vi "TCP Engine Send Commands To all Modules.vi"(6 "Main Engine Command Q":refnum<queue>, 7 "Active Engine Names":string[](array[string]), 8 "error in":errorcluster, 9 "Engine Name":string[](array[string]), 10 "TCP Engine Log File Path":path, 11 "JSON String":string) -> (0 "error out":errorcluster, 3 "Active Engine Names Out":string[](array[string]))   [LabVIEW 2024, in "TCP Engine.lvlib"]
doc: "The purpose of this VI is to perform all functions of the hardware modules.\nFunctions\n1)Engine Launch\n2)Configuration\n3)Update\n4)All Start\n5)Engine start\n6)Hardware Info.\n\n\nAll Rights Reserved © 2017 SyncSols"
uses:
  TCP Engine.lvlib
  Main Engine/Controls/Main Engine Command Cluster.ctl
  Main Engine/Controls/Main Engine TCP Command Data.ctl
  Analog Output/Controls/AO JSON Data Cluster.ctl
  Analog Output/Controls/AO Interface Data Cluster.ctl
  Analog Output/Controls/AO Channel Configuration Cluster.ctl
  Analog Output/Controls/AO Timing Cluster.ctl
  Analog Output/Controls/AIO Command Q Cluster.ctl
  Main Engine/Controls/Main Engine JSON Command State.ctl
  Controls/TCP Engine I&O  Interupt Cluster.ctl
  Analog Output/Controls/AO 1D DBL ArrayCluster.ctl
  Analog Output/Controls/AO 1D DBL Interface Data Cluster.ctl
  Analog Output/Controls/AO DBL Data Cluster.ctl
  Digital Output/Controls/DIO Configuration cluster.ctl
  Digital Output/Controls/DIO Interface Data.ctl
  Digital Output/SubVIs/Digital Dynamic Cluster.ctl
  Digital Output/Controls/DIO Commad Q Cluster.ctl
  Digital Output/Controls/DO Update Cluster.ctl
  Async Serial/Controls/Async Serial Command Q Cluster.ctl
  Async Serial/Controls/Async Serial Configuration Cluster.ctl
  Async Serial/Controls/Async Frame Info Cluster.ctl
  Async Serial/Controls/Async Message Info Cluster.ctl
  Controls/TCP Engine Serial Interupt Cluster.ctl
  Async Serial/Controls/Async Update Cluster.ctl
  Async Serial/Controls/Async Waveform Config Cluster.ctl
  Analog Output/Controls/AO Sampling Info Cluster.ctl
  Ethernet/Controls/Ethernet Command Q Cluster.ctl
  Ethernet/Controls/Ethernet Configuration Cluster.ctl
  Ethernet/Controls/Ethernet Frame Info Cluster.ctl
  Ethernet/Controls/Ethernet Message Info Cluster.ctl
  Ethernet/Controls/Ethernet Dynamic Data Cluster.ctl
  Ethernet/Controls/Ethernet Update Cluster.ctl
  Controls/TCP Engine Q Driver Options.ctl
  Controls/TCP Engine State Machine Cases.ctl
  <vilib>/Utility/error.llb/Error Cluster From Error Code.vi
  <vilib>/ErrorRing/Error Ring.xnode
  <vilib>/addons/_JKI.lib/Serialization/JSON/JKI JSON Serialization.lvlib
  RT-DQMH-Module's/RT-AutoSequence/RT-AutoSequence.lvlib
  RT-DQMH-Module's/RT-TDMS-Logging/RT-TDMS-Logging.lvlib
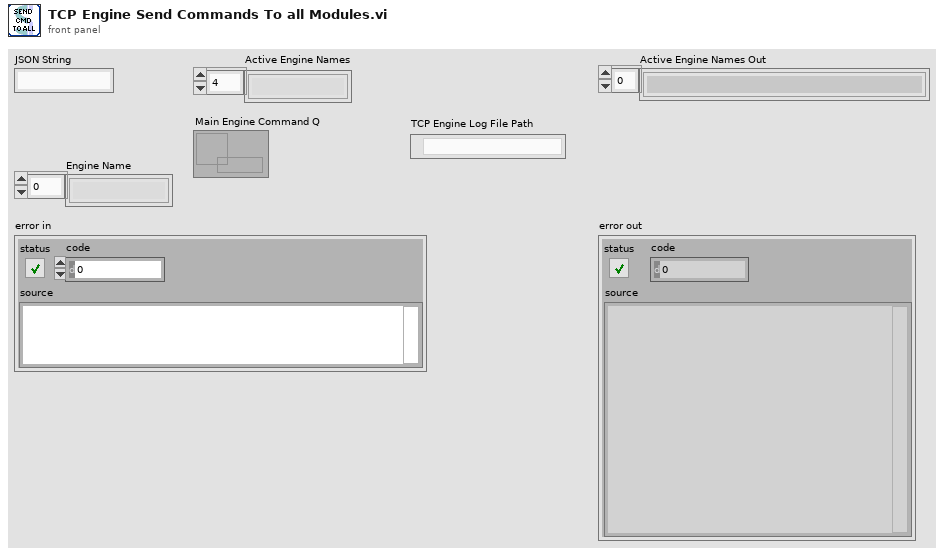
[diagram p1: front panel]
types:
  T1 = typedef "Main Engine TCP Command Data.ctl" = enum16{"Get HW Info", "Launch Module", "Get CPU Load", "Close CPU Load", "Exit"}
  T2 = typedef "Main Engine Command Cluster.ctl" = cluster{"State":T1, "Interface":string, "Engine Name":string, "Varient Data":variant, "SubCmd":string, "Serial Mode":string, "ARINC Board":u8, "Ethernet Mode":u8, "CPU Frequency":dbl}
  T3 = typedef "Main Engine JSON Command State.ctl" = enum16{"Configure", "Start", "Exit"}
  T4 = typedef "AO JSON Data Cluster.ctl" = cluster{"Interface":string, "Interface Data":T5}
  T5 = typedef "AO Interface Data Cluster.ctl" = cluster{"Command":string, "SubCmd":string, "Data":T6[], "Timing":T7}
  T6 = typedef "AO Channel Configuration Cluster.ctl" = cluster{"Channel":string, "Min Value":dbl, "Max Value":dbl, "Type":string, "Terminal Configure":u16, "Dynamic":u8, "Dyn Type":string, "Data":dbl[], "File Name":string, "Column":i32, "Frequency":dbl}
  T7 = typedef "AO Timing Cluster.ctl" = cluster{"samples per channel":i32, "sample mode":i32, "Sampling Rate":dbl}
  T8 = typedef "AIO Command Q Cluster.ctl" = cluster{"Interface":string, "Interface Data":T5, "Command State":T3}
  T9 = typedef "AO 1D DBL ArrayCluster.ctl" = cluster{"Interface":string, "Interface Data":T10}
  T10 = typedef "AO 1D DBL Interface Data Cluster.ctl" = cluster{"Command":string, "SubCmd":string, "Data":T11[]}
  T11 = typedef "AO DBL Data Cluster.ctl" = cluster{"Channel":string, "Data":dbl}
  T12 = typedef "DIO Commad Q Cluster.ctl" = cluster{"Interface":string, "Interface Data":cluster{"Command":string, "SubCmd":string, "Frequency":u16, "Data":T13[]}, "Command State":T3, "Data":variant}
  T13 = typedef "Digital Dynamic Cluster.ctl" = cluster{"Channel":string, "Data":u8[], "Identification Name":string}
  T14 = typedef "DO Update Cluster.ctl" = cluster{"Channel":string[], "Data":u8[]}
  T15 = typedef "Async Serial Configuration Cluster.ctl" = cluster{"Port":string, "Minor Frame Freq":u16, "Minor Frame Count":u16, "Frame Info":T16[], "Sensor Type":u16, "OIM Address":u16}
  T16 = typedef "Async Frame Info Cluster.ctl" = cluster{"Frame ID":u16, "Message Info":T17[]}
  T17 = typedef "Async Message Info Cluster.ctl" = cluster{"Message":u8[], "Message Name":string}
  T18 = typedef "Async Serial Command Q Cluster.ctl" = cluster{"Async serial Configuration Cluster":T15, "Command State":T3}
  T19 = typedef "Async Update Cluster.ctl" = cluster{"Port":string, "Message Info":T17[]}
  T20 = typedef "Async Waveform Config Cluster.ctl" = cluster{"Port":string, "Pattern":string, "Amplitude":dbl, "Frequency":dbl, "Phase":i32, "Sampling info":T21}
  T21 = typedef "AO Sampling Info Cluster.ctl" = cluster{"Fs":dbl, "#s":dbl}
  T22 = typedef "Ethernet Configuration Cluster.ctl" = cluster{"Mode":u8, "Local IP":string, "Local Port":u16, "Frame Info":T23[], "Minor Frame Freq":u8}
  T23 = typedef "Ethernet Frame Info Cluster.ctl" = cluster{"Frame ID":u16, "Message Info":T24[]}
  T24 = typedef "Ethernet Message Info Cluster.ctl" = cluster{"Message":u8[], "Message Name":string, "Dynamic":u8, "DynData":T25[], "Client IP":string, "Client Port":u16}
  T25 = typedef "Ethernet Dynamic Data Cluster.ctl" = cluster{"Type":string, "Start Byte":u8, "End Byte":u8, "Data":u32[][], "File Name":string, "Column":i32}
  T26 = typedef "Ethernet Command Q Cluster.ctl" = cluster{"Ethernet Configuration":T22, "Command State":T3}
  T27 = typedef "Ethernet Update Cluster.ctl" = cluster{"IP":string, "Message Info":T17[], "Port":u16}
  T28 = typedef "TCP Engine.lvlib/TCP Engine Q Driver Options.ctl" = enum16{"Initialize", "EnQ", "DeQ", "EnQ at Opp", "Get Q Status", "Flush Q", "Release Q"}
  T29 = typedef "TCP Engine.lvlib/TCP Engine I&O  Interupt Cluster.ctl" = cluster{" Stop":bool, "JSON Variant":variant}
  T30 = typedef "DIO Configuration cluster.ctl" = cluster{"Interface":string, "Interface Data":T31}
  T31 = typedef "DIO Interface Data.ctl" = cluster{"Command":string, "SubCmd":string, "Frequency":u16, "Data":T13[]}
  T32 = typedef "TCP Engine.lvlib/TCP Engine Serial Interupt Cluster.ctl" = cluster{"Stop":bool, "JSON Variant":variant}
  T33 = typedef "TCP Engine.lvlib/TCP Engine State Machine Cases.ctl" = enum16{">Poll", ".........State Machine.........", ">Init", ">Init Configuration", ">Decode Configuration", ">Error", ">Exit", "..........TCP Engine..........", ">Wait for Listener", ">Get Msg from HOST", ">Decode the Command", ">Create Listerner ID"}
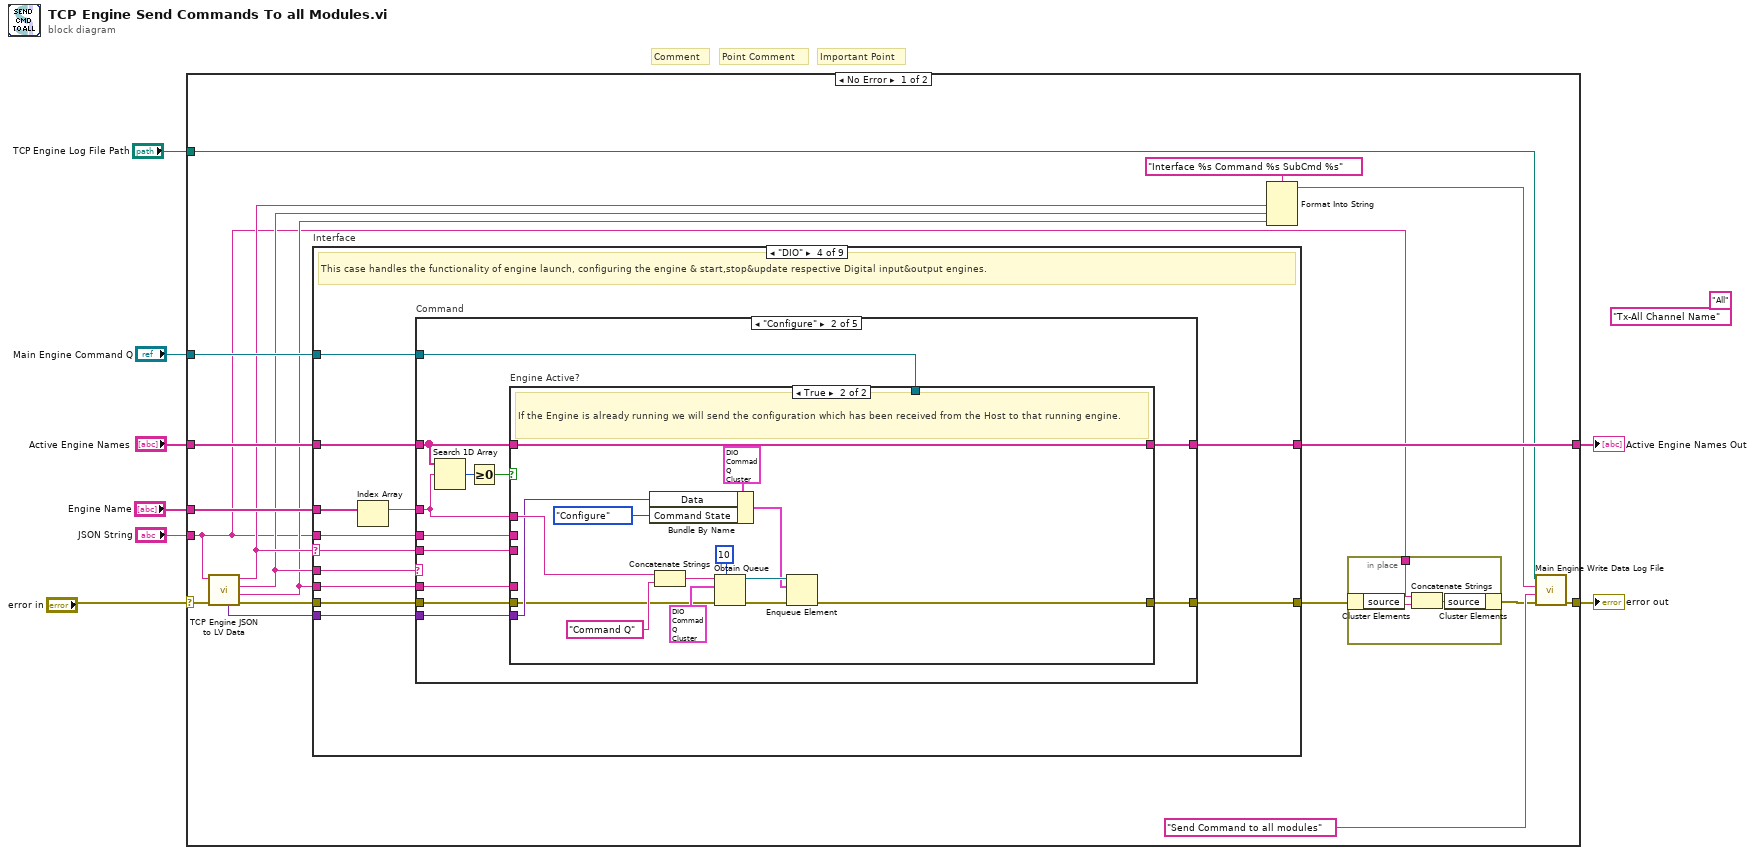
[diagram p0: block diagram]
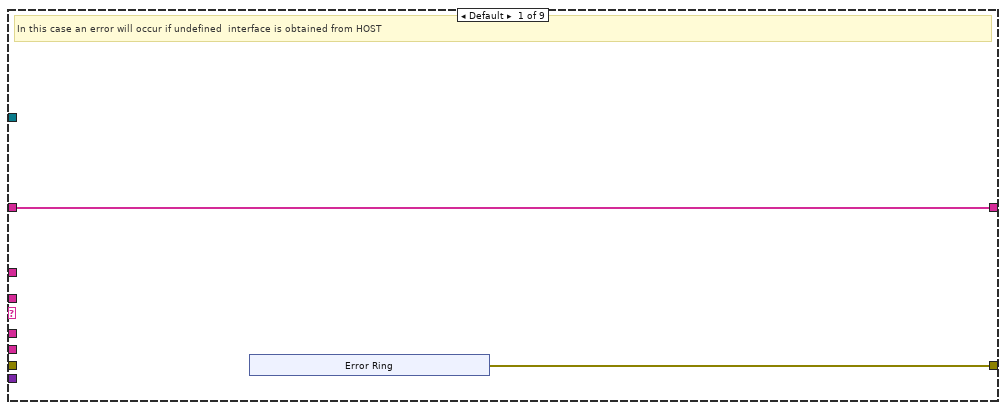
[diagram p2: hidden frame]
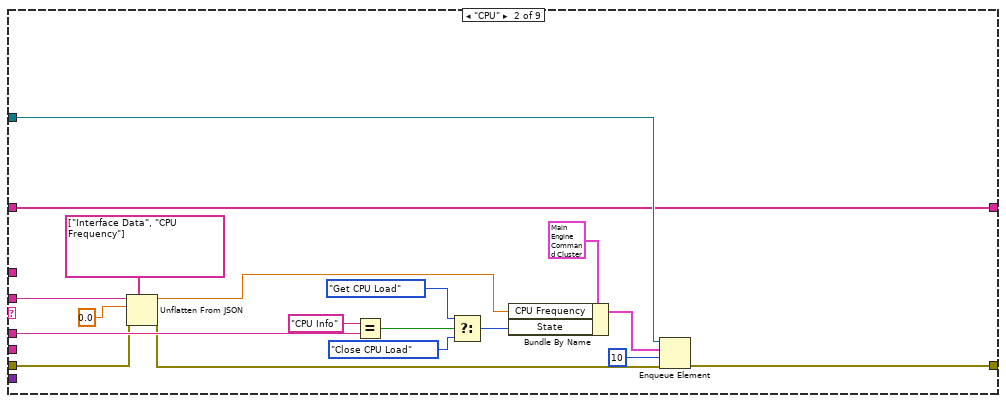
[diagram p3: hidden frame]
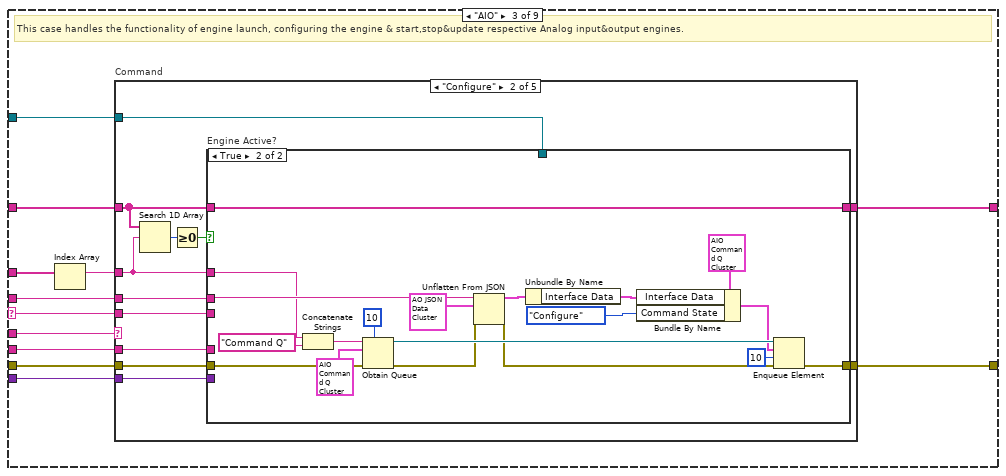
[diagram p4: hidden frame]
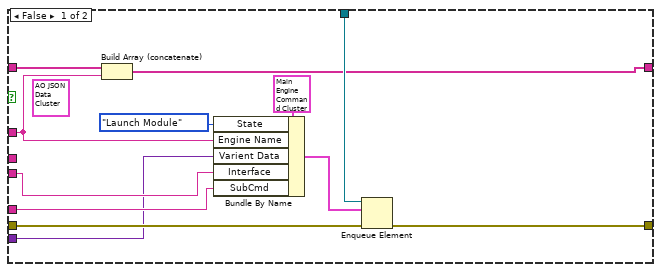
[diagram p6: hidden frame]
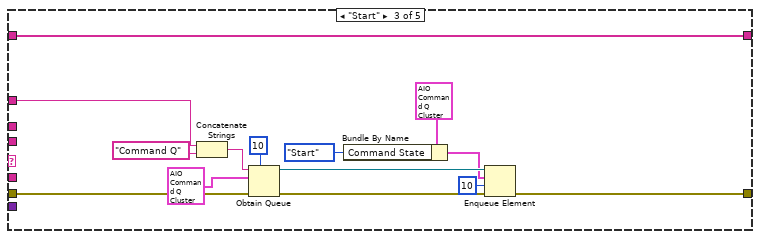
[diagram p7: hidden frame]
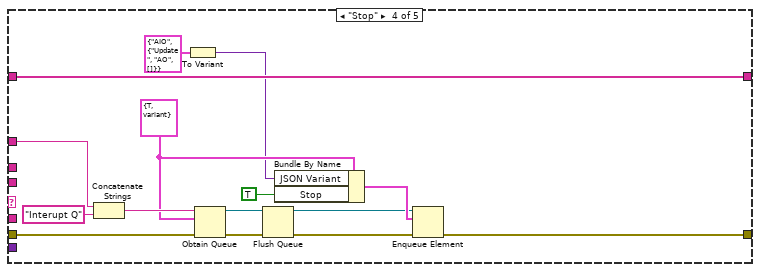
[diagram p8: hidden frame]
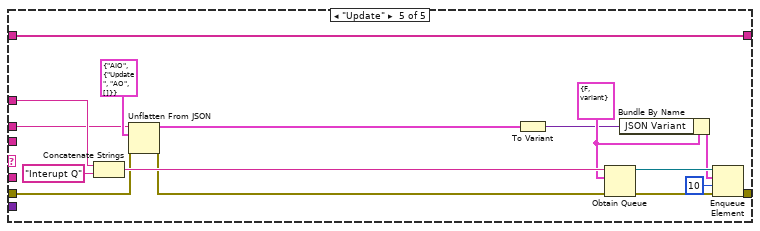
[diagram p9: hidden frame]
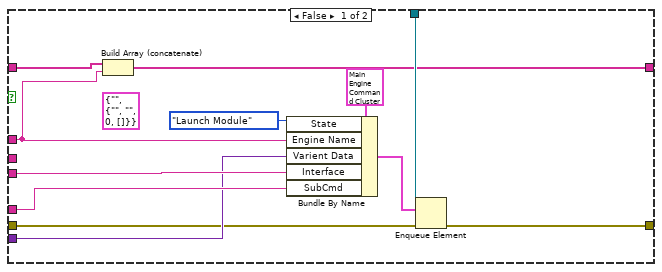
[diagram p11: hidden frame]
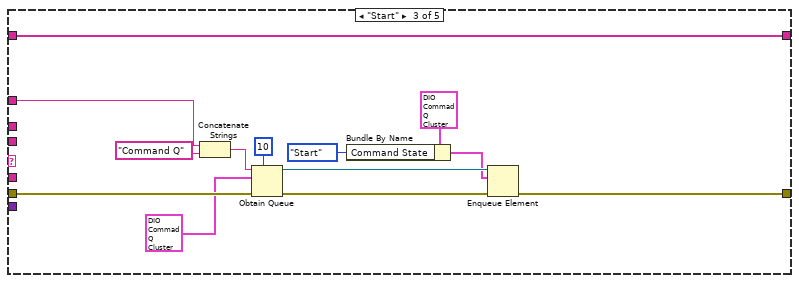
[diagram p12: hidden frame]
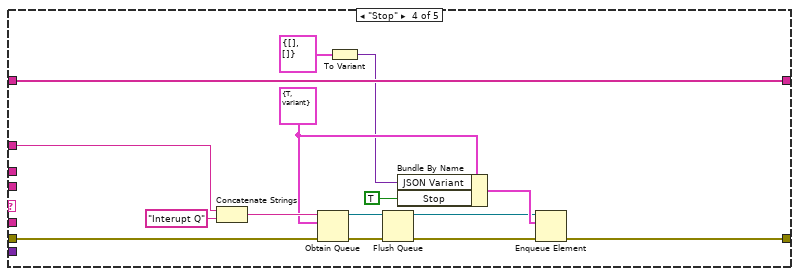
[diagram p13: hidden frame]
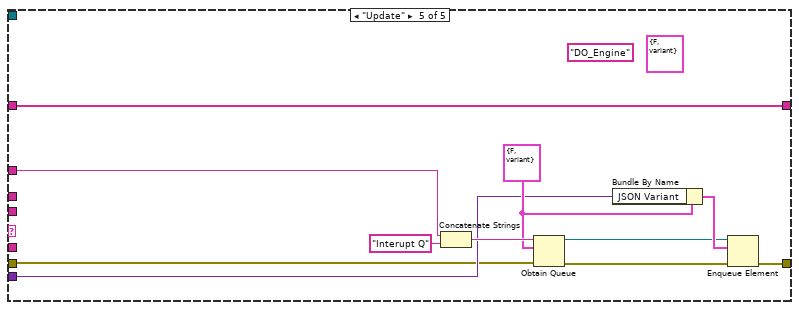
[diagram p14: hidden frame]
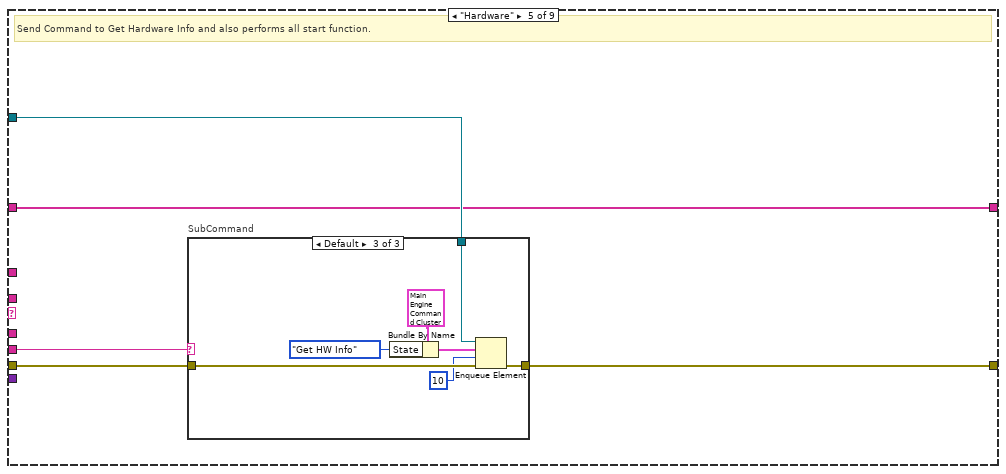
[diagram p15: hidden frame]
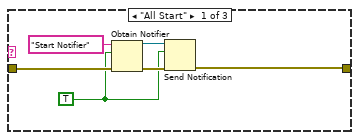
[diagram p16: hidden frame]
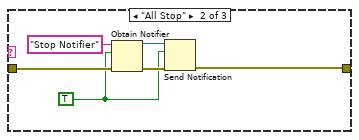
[diagram p17: hidden frame]
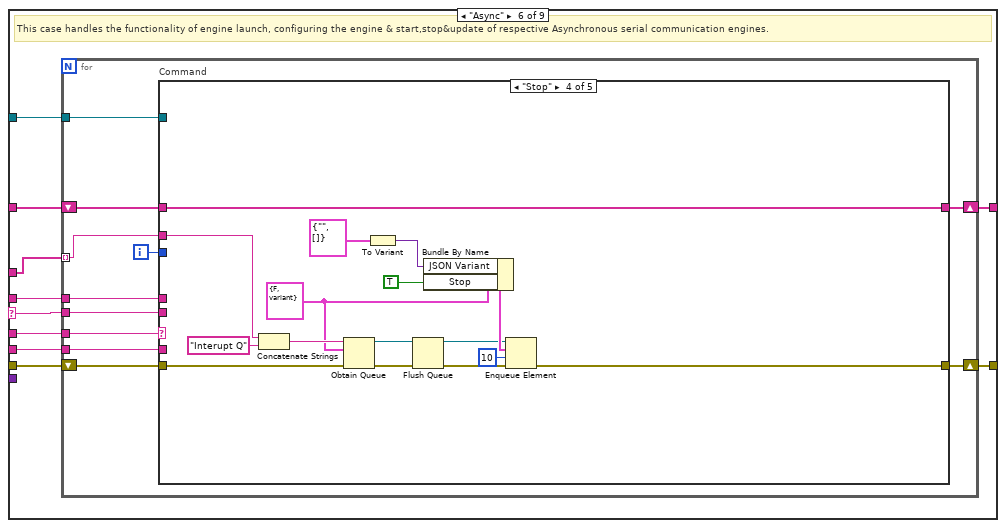
[diagram p18: hidden frame]
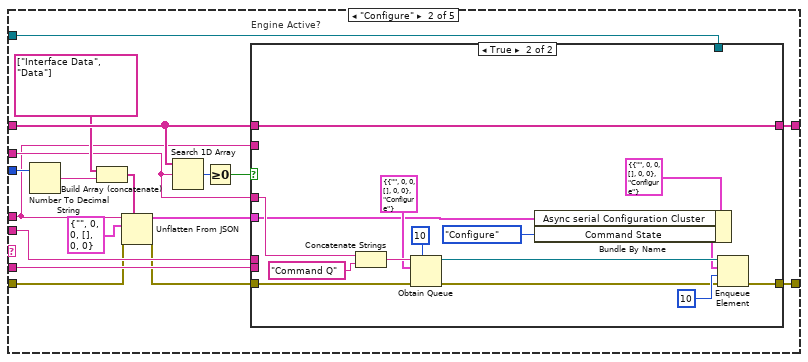
[diagram p20: hidden frame]
diagram:
  (unwired) "Tx-All Channel Name" ("Interface Data.Command")
  (unwired) "All" ("Interface")
  # "Important Point"
  # "Point Comment"
  # "Comment"
  n1 = case shown="No Error" "error in" {
    selector: "error in" -> [w24 w610]
    tunnel: [w20 w612] -> w8
    tunnel: "Engine Name" -> [w22 _]
    tunnel: "JSON String" -> [w10 w609]
    tunnel: "Main Engine Command Q" -> [w26 _]
    tunnel: "Active Engine Names" -> [w25 w613]
    tunnel: [w21 w613] -> w3
    tunnel: "TCP Engine Log File Path" -> [w14 w611]
    frame No Error {
      n2 = call "TCP Engine JSON to LV Data.vi"("error in"=w24, "Cmd String"=w10) -> ("error out"=w23:errorcluster, "SubCmd"=w16:string, "Command"=w17:string, "Interface"=w18:string, "Data"=w9:variant)  [unwired: 4 in, 1 out]
      n3 = case "Interface" shown="\"DIO\"" w18 {
        selector: w18 -> [_ _ w58 w160 _ w276 w421 _ _]
        tunnel: [w31 w54 w64 w166 w250 w281 w426 w548 w579] -> w12
        tunnel: w23 -> [_ w42 w66 w168 w252 w274 w419 w544 w578]
        tunnel: w26 -> [_ w53 w65 w167 w251 w279 w424 _ _]
        tunnel: w22 -> [_ _ w63 w165 _ w275 w420 _ _]
        tunnel: w10 -> [_ w40 w62 w164 _ w273 w418 _ _]
        tunnel: w25 -> [w30 w43 w60 w162 w249 w278 w423 w545 w581]
        tunnel: w17 -> [_ w49 w61 w163 _ w272 w417 _ w580]
        tunnel: w16 -> [_ _ w59 w161 w248 w277 w422 _ w577]
        tunnel: [w30 w43 w57 w159 w249 w280 w425 w545 w581] -> w21
        tunnel: w9 -> [_ _ w55 w157 _ _ _ _ w576]
        frame Default {
          # "In this case an error will occur if undefined  interface is obtained from HOST"
          n4 = xnode "Error Ring"() -> ("error out"=w31:errorcluster)
        }
        frame "CPU" {
          n5 = Unflatten From JSON(path=string[] ["Interface Data", "CPU Frequency"], JSON string=w40, type and defaults=0.0, error in (no error)=w42) -> (value=w37:dbl, error out=w41:errorcluster)  [unwired: 3 in]
          n6 = Equal?(x="CPU Info", y=w49) -> (x = y?=w47:bool)
          n7 = Select(t=Main_Engine_TCP_Command_Data."Get CPU Load" ("State"), s=w47, f=Main_Engine_TCP_Command_Data."Close CPU Load" ("State")) -> (s? t:f=w44:T1)
          n8 = Bundle By Name(cluster=T2 {"State"=enum."Launch Module", "Interface"="AO", "Engine Name"="Slot5_6551_AO", "Varient Data"=variant(string "{"), "SubCmd"="", "Serial Mode"="", "ARINC Board"=0, "Ethernet Mode"=0, "CPU Frequency"=0.0}, "CPU Frequency"=w37, "State"=w44) -> (w50:T2)
          n9 = Enqueue Element(queue=w53, element=w50, timeout in ms (-1)=10, error in (no error)=w41) -> (error out=w54:errorcluster)  [unwired: 2 out]
        }
        frame "AIO" {
          # "This case handles the functionality of engine launch, configuring the engine & start,stop&update respective Analog input&output engines."
          n10 = Index Array(array=w63) -> (element=w56:string)  [unwired: 1 in]
          n11 = case "Command" shown="\"Configure\"" w61 {
            tunnel: w66 -> [w68 w80 w125 w140 w146]
            tunnel: w65 -> [_ w79 _ _ _]
            tunnel: [w68 w78 w124 w133 w149] -> w64
            tunnel: w56 -> [_ w70 w123 w138 w155]
            tunnel: w62 -> [_ w77 _ _ w144]
            tunnel: w60 -> [w67 w72 w112 w132 w148]
            tunnel: w59 -> [_ w74 _ _ _]
            tunnel: w58 -> [_ w73 _ _ _]
            tunnel: [w67 w71 w112 w132 w148] -> w57
            tunnel: w55 -> [_ w69 _ _ _]
            frame Default {
            }
            frame "Configure" {
              n12 = Search 1D Array(1D array=w72, element=w70) -> (index of element=w76:i32)  [unwired: 1 in]
              n13 = Greater Or Equal To 0?(x=w76) -> (x >= 0?=w75:bool)
              n14 = case "Engine Active?" shown="True" w75 {
                tunnel: w80 -> [w92 w111]
                tunnel: w79 -> [w91 _]
                tunnel: [w90 w110] -> w78
                tunnel: w77 -> [_ w95]
                tunnel: w74 -> [w83 _]
                tunnel: w73 -> [w86 _]
                tunnel: w72 -> [w85 w93]
                tunnel: [w84 w93] -> w71
                tunnel: w70 -> [w82 w94]
                tunnel: w69 -> [w81 _]
                frame False {
                  (unwired) T4 {"Interface"="AIO", "Interface Data"={"Command"="Configure", "SubCmd"="AO", "Data"=[], "Timing"={"samples per channel"=0, "sample mode"=10178, "Sampling Rate"=0.0}}} ("AO JSON Data Cluster")
                  n15 = Build Array (concatenate)(w85, w82) -> (w84:string[])
                  n16 = Bundle By Name(cluster=T2 {"State"=enum."Launch Module", "Interface"="AO", "Engine Name"="Slot5_6551_AO", "Varient Data"=variant(string "{"), "SubCmd"="", "Serial Mode"="", "ARINC Board"=0, "Ethernet Mode"=0, "CPU Frequency"=0.0}, "State"=Main_Engine_TCP_Command_Data."Launch Module", "Engine Name"=w82, "Varient Data"=w81, "Interface"=w86, "SubCmd"=w83) -> (w88:T2)
                  n17 = Enqueue Element(queue=w91, element=w88, error in (no error)=w92) -> (error out=w90:errorcluster)  [unwired: 1 in, 2 out]
                }
                frame True {
                  n18 = Concatenate Strings(w94, "Command Q" ("string")) -> (w109:string)
                  n19 = Obtain Queue(max queue size (-1, unlimited)=10, name (unnamed)=w109, element data type=T8 {"Interface"="AIO", "Interface Data"={"Command"="Configure", "SubCmd"="AO", "Data"=[], "Timing"={"samples per channel"=1000, "sample mode"=10178, "Sampling Rate"=1000.0}}, "Command State"=enum."Configure"}, error in (no error)=w111) -> (queue out=w107:refnum<queue>, error out=w97:errorcluster)  [unwired: 1 in, 1 out]
                  n20 = Unflatten From JSON(JSON string=w95, type and defaults=T4 {"Interface"="AIO", "Interface Data"={"Command"="Configure", "SubCmd"="AO", "Data"=[], "Timing"={"samples per channel"=1000, "sample mode"=10178, "Sampling Rate"=1000.0}}}, error in (no error)=w97) -> (value=w101:T4, error out=w96:errorcluster)  [unwired: 4 in]
                  n21 = Unbundle By Name(w101) -> ("Interface Data"=w100:T5)
                  n22 = Bundle By Name(cluster=T8 {"Interface"="AIO", "Interface Data"={"Command"="Configure", "SubCmd"="AO", "Data"=[], "Timing"={"samples per channel"=1000, "sample mode"=10178, "Sampling Rate"=1000.0}}, "Command State"=enum."Configure"}, "Interface Data"=w100, "Command State"=Main_Engine_JSON_Command_State."Configure") -> (w98:T8)
                  n23 = Enqueue Element(queue=w107, element=w98, timeout in ms (-1)=10, error in (no error)=w96) -> (error out=w110:errorcluster)  [unwired: 2 out]
                }
              }
            }
            frame "Start" {
              n24 = Concatenate Strings(w123, "Command Q" ("string")) -> (w122:string)
              n25 = Obtain Queue(max queue size (-1, unlimited)=10, name (unnamed)=w122, element data type=T8 {"Interface"="AIO", "Interface Data"={"Command"="Configure", "SubCmd"="AO", "Data"=[], "Timing"={"samples per channel"=1000, "sample mode"=10178, "Sampling Rate"=1000.0}}, "Command State"=enum."Configure"}, error in (no error)=w125) -> (queue out=w120:refnum<queue>, error out=w113:errorcluster)  [unwired: 1 in, 1 out]
              n26 = Bundle By Name(cluster=T8 {"Interface"="AIO", "Interface Data"={"Command"="Configure", "SubCmd"="AO", "Data"=[], "Timing"={"samples per channel"=1000, "sample mode"=10178, "Sampling Rate"=1000.0}}, "Command State"=enum."Configure"}, "Command State"=Main_Engine_JSON_Command_State."Start") -> (w114:T8)
              n27 = Enqueue Element(queue=w120, element=w114, timeout in ms (-1)=10, error in (no error)=w113) -> (error out=w124:errorcluster)  [unwired: 2 out]
            }
            frame "Stop" {
              w136 = T29 {" Stop"=TRUE, "JSON Variant"=variant(string "")} ("I/O  Interupt Cluster")
              n28 = Concatenate Strings(w138, "Interupt Q" ("string")) -> (w139:string)
              n29 = To Variant(anything=T9 {"Interface"="AIO", "Interface Data"={"Command"="Update", "SubCmd"="AO", "Data"=[]}}) -> (Variant=w126:variant)
              n30 = Obtain Queue(name (unnamed)=w139, element data type=w136, error in (no error)=w140) -> (queue out=w131:refnum<queue>, error out=w129:errorcluster)  [unwired: 2 in, 1 out]
              n31 = Flush Queue(queue=w131, error in (no error)=w129) -> (queue out=w130:refnum<queue>, error out=w128:errorcluster)  [unwired: 1 out]
              n32 = Bundle By Name(cluster=w136, "JSON Variant"=w126, "Stop"=TRUE ("Generation Stop")) -> (w134:T29)
              n33 = Enqueue Element(queue=w130, element=w134, error in (no error)=w128) -> (error out=w133:errorcluster)  [unwired: 1 in, 2 out]
            }
            frame "Update" {
              w151 = T29 {" Stop"=FALSE, "JSON Variant"=variant(string "")} ("I/O  Interupt Cluster")
              n34 = Concatenate Strings(w155, "Interupt Q" ("string")) -> (w156:string)
              n35 = Unflatten From JSON(JSON string=w144, type and defaults=T9 {"Interface"="AIO", "Interface Data"={"Command"="Update", "SubCmd"="AO", "Data"=[]}}, error in (no error)=w146) -> (value=w141:T9, error out=w143:errorcluster)  [unwired: 4 in]
              n36 = To Variant(anything=w141) -> (Variant=w147:variant)
              n37 = Obtain Queue(name (unnamed)=w156, element data type=w151, error in (no error)=w143) -> (queue out=w153:refnum<queue>, error out=w152:errorcluster)  [unwired: 2 in, 1 out]
              n38 = Bundle By Name(cluster=w151, "JSON Variant"=w147) -> (w150:T29)
              n39 = Enqueue Element(queue=w153, element=w150, timeout in ms (-1)=10, error in (no error)=w152) -> (error out=w149:errorcluster)  [unwired: 2 out]
            }
          }
        }
        frame "DIO" {
          # "This case handles the functionality of engine launch, configuring the engine & start,stop&update respective Digital input&output engines."
          n40 = Index Array(array=w165) -> (element=w158:string)  [unwired: 1 in]
          n41 = case "Command" shown="\"Configure\"" w163 {
            tunnel: w168 -> [w170 w182 w221 w236 w239]
            tunnel: w167 -> [_ w181 _ _ _]
            tunnel: [w170 w180 w220 w229 w242] -> w166
            tunnel: w158 -> [_ w172 w219 w234 w238]
            tunnel: w164 -> [_ w179 _ _ _]
            tunnel: w162 -> [w169 w174 w210 w228 w241]
            tunnel: w161 -> [_ w176 _ _ _]
            tunnel: w160 -> [_ w175 _ _ _]
            tunnel: [w169 w173 w210 w228 w241] -> w159
            tunnel: w157 -> [_ w171 _ _ w240]
            frame Default {
            }
            frame "Configure" {
              n42 = Search 1D Array(1D array=w174, element=w172) -> (index of element=w178:i32)  [unwired: 1 in]
              n43 = Greater Or Equal To 0?(x=w178) -> (x >= 0?=w177:bool)
              n44 = case "Engine Active?" shown="True" w177 {
                tunnel: w182 -> [w183 w195]
                tunnel: w181 -> [w194 _]
                tunnel: [w193 w208] -> w180
                tunnel: w179 -> [_ _]
                tunnel: w176 -> [w186 _]
                tunnel: w175 -> [w189 _]
                tunnel: w174 -> [w188 w198]
                tunnel: [w187 w198] -> w173
                tunnel: w172 -> [w185 w199]
                tunnel: w171 -> [w184 w196]
                frame False {
                  (unwired) T30 {"Interface"="", "Interface Data"={"Command"="", "SubCmd"="", "Frequency"=0, "Data"=[]}} ("DIO Configuration Cluster")
                  n45 = Build Array (concatenate)(w188, w185) -> (w187:string[])
                  n46 = Bundle By Name(cluster=T2 {"State"=enum."Launch Module", "Interface"="AO", "Engine Name"="Slot5_6551_AO", "Varient Data"=variant(string "{"), "SubCmd"="", "Serial Mode"="", "ARINC Board"=0, "Ethernet Mode"=0, "CPU Frequency"=0.0}, "State"=Main_Engine_TCP_Command_Data."Launch Module", "Engine Name"=w185, "Varient Data"=w184, "Interface"=w189, "SubCmd"=w186) -> (w191:T2)
                  n47 = Enqueue Element(queue=w194, element=w191, error in (no error)=w183) -> (error out=w193:errorcluster)  [unwired: 1 in, 2 out]
                }
                frame True {
                  # "If the Engine is already running we will send the configuration which has been received from the Host to that running engine."
                  n48 = Bundle By Name(cluster=T12 {"Interface"="AIO", "Interface Data"={"Command"="Configure", "SubCmd"="AO", "Frequency"=0, "Data"=[]}, "Command State"=enum."Configure", "Data"=variant}, "Data"=w196, "Command State"=Main_Engine_JSON_Command_State."Configure") -> (w201:T12)
                  n49 = Concatenate Strings(w199, "Command Q" ("string")) -> (w207:string)
                  n50 = Obtain Queue(max queue size (-1, unlimited)=10, name (unnamed)=w207, element data type=T12 {"Interface"="AIO", "Interface Data"={"Command"="Configure", "SubCmd"="AO", "Frequency"=0, "Data"=[]}, "Command State"=enum."Configure", "Data"=variant}, error in (no error)=w195) -> (queue out=w205:refnum<queue>, error out=w197:errorcluster)  [unwired: 1 in, 1 out]
                  n51 = Enqueue Element(queue=w205, element=w201, error in (no error)=w197) -> (error out=w208:errorcluster)  [unwired: 1 in, 2 out]
                }
              }
            }
            frame "Start" {
              n52 = Concatenate Strings(w219, "Command Q" ("string")) -> (w218:string)
              n53 = Obtain Queue(max queue size (-1, unlimited)=10, name (unnamed)=w218, element data type=T12 {"Interface"="AIO", "Interface Data"={"Command"="Configure", "SubCmd"="AO", "Frequency"=0, "Data"=[]}, "Command State"=enum."Configure", "Data"=variant}, error in (no error)=w221) -> (queue out=w216:refnum<queue>, error out=w213:errorcluster)  [unwired: 1 in, 1 out]
              n54 = Bundle By Name(cluster=T12 {"Interface"="AIO", "Interface Data"={"Command"="Configure", "SubCmd"="AO", "Frequency"=0, "Data"=[]}, "Command State"=enum."Configure", "Data"=variant}, "Command State"=Main_Engine_JSON_Command_State."Start") -> (w214:T12)
              n55 = Enqueue Element(queue=w216, element=w214, error in (no error)=w213) -> (error out=w220:errorcluster)  [unwired: 1 in, 2 out]
            }
            frame "Stop" {
              w232 = T29 {" Stop"=TRUE, "JSON Variant"=variant(string "")} ("I/O  Interupt Cluster")
              n56 = Concatenate Strings(w234, "Interupt Q" ("string")) -> (w235:string)
              n57 = Obtain Queue(name (unnamed)=w235, element data type=w232, error in (no error)=w236) -> (queue out=w227:refnum<queue>, error out=w225:errorcluster)  [unwired: 2 in, 1 out]
              n58 = To Variant(anything=T14 {"Channel"=[], "Data"=[]}) -> (Variant=w222:variant)
              n59 = Flush Queue(queue=w227, error in (no error)=w225) -> (queue out=w226:refnum<queue>, error out=w224:errorcluster)  [unwired: 1 out]
              n60 = Bundle By Name(cluster=w232, "JSON Variant"=w222, "Stop"=TRUE ("Generation Stop")) -> (w230:T29)
              n61 = Enqueue Element(queue=w226, element=w230, error in (no error)=w224) -> (error out=w229:errorcluster)  [unwired: 1 in, 2 out]
            }
            frame "Update" {
              (unwired) T29 {" Stop"=FALSE, "JSON Variant"=variant(string "")} ("I/O  Interupt Cluster")
              (unwired) "DO_Engine" ("Engine Name")
              w244 = T29 {" Stop"=FALSE, "JSON Variant"=variant(string "")} ("I/O  Interupt Cluster")
              n62 = Concatenate Strings(w238, "Interupt Q" ("string")) -> (w247:string)
              n63 = Obtain Queue(name (unnamed)=w247, element data type=w244, error in (no error)=w239) -> (queue out=w237:refnum<queue>, error out=w245:errorcluster)  [unwired: 2 in, 1 out]
              n64 = Bundle By Name(cluster=w244, "JSON Variant"=w240) -> (w243:T29)
              n65 = Enqueue Element(queue=w237, element=w243, error in (no error)=w245) -> (error out=w242:errorcluster)  [unwired: 1 in, 2 out]
            }
          }
        }
        frame "Hardware" {
          # "Send Command to Get Hardware Info and also performs all start function."
          n66 = case "SubCommand" shown="Default" w248 {
            tunnel: w252 -> [w256 w262 w271]
            tunnel: w251 -> [_ _ w270]
            tunnel: [w258 w264 w269] -> w250
            frame "All Start" {
              w253 = TRUE
              n67 = Obtain Notifier(name (unnamed)="Start Notifier", notification data type=w253, error in (no error)=w256) -> (notifier out=w254:refnum<notifier>, error out=w257:errorcluster)  [unwired: 1 in, 1 out]
              n68 = Send Notification(notification=w253, notifier=w254, error in (no error)=w257) -> (error out=w258:errorcluster)  [unwired: 1 out]
            }
            frame "All Stop" {
              w259 = TRUE
              n69 = Obtain Notifier(name (unnamed)="Stop Notifier", notification data type=w259, error in (no error)=w262) -> (notifier out=w260:refnum<notifier>, error out=w263:errorcluster)  [unwired: 1 in, 1 out]
              n70 = Send Notification(notification=w259, notifier=w260, error in (no error)=w263) -> (error out=w264:errorcluster)  [unwired: 1 out]
            }
            frame Default {
              n71 = Bundle By Name(cluster=T2 {"State"=enum."Launch Module", "Interface"="AO", "Engine Name"="Slot5_6551_AO", "Varient Data"=variant(string "{"), "SubCmd"="", "Serial Mode"="", "ARINC Board"=0, "Ethernet Mode"=0, "CPU Frequency"=0.0}, "State"=Main_Engine_TCP_Command_Data."Get HW Info") -> (w266:T2)
              n72 = Enqueue Element(queue=w270, element=w266, timeout in ms (-1)=10, error in (no error)=w271) -> (error out=w269:errorcluster)  [unwired: 2 out]
            }
          }
        }
        frame "Async" {
          # "This case handles the functionality of engine launch, configuring the engine & start,stop&update of respective Asynchronous serial communication engines."
          n73 = for {
            tunnel: w279 -> [w290]
            tunnel: w277 -> [w288]
            tunnel: w276 -> [w287]
            tunnel: w272 -> [w286]
            tunnel: w275 -> [w282] mode=indexing
            shift-right: [w292] -> w281
            shift-left: w274 -> [w284]
            tunnel: w273 -> [w285]
            shift-right: [w291] -> w280
            shift-left: w278 -> [w289]
            i -> [w283]
            n74 = case "Command" shown="\"Stop\"" w286 {
              tunnel: w284 -> [w294 w300 w359 w375 w387]
              tunnel: w290 -> [_ w312 _ _ _]
              tunnel: [w294 w311 w358 w370 w393] -> w292
              tunnel: w289 -> [w293 w306 w347 w369 w392]
              tunnel: w288 -> [_ w308 _ _ _]
              tunnel: w287 -> [_ w307 _ _ _]
              tunnel: [w293 w305 w347 w369 w392] -> w291
              tunnel: w285 -> [_ w295 _ _ w381]
              tunnel: w283 -> [_ w304 _ _ w391]
              tunnel: w282 -> [_ w297 w346 w368 w386]
              frame Default {
              }
              frame "Configure" {
                n75 = Number To Decimal String(number=w304) -> (decimal integer string=w302:string)  [unwired: 1 in]
                n76 = Build Array (concatenate)(string[] ["Interface Data", "Data"] ("path"), w302) -> (w298:string[])
                n77 = Unflatten From JSON(path=w298, JSON string=w295, type and defaults=T15 {"Port"="", "Minor Frame Freq"=0, "Minor Frame Count"=0, "Frame Info"=[], "Sensor Type"=0, "OIM Address"=0} ("Array"), error in (no error)=w300) -> (value=w296:T15, error out=w299:errorcluster)  [unwired: 3 in]
                n78 = Search 1D Array(1D array=w306, element=w297) -> (index of element=w310:i32)  [unwired: 1 in]
                n79 = Greater Or Equal To 0?(x=w310) -> (x >= 0?=w309:bool)
                n80 = case "Engine Active?" shown="True" w309 {
                  tunnel: w312 -> [w330 _]
                  tunnel: [w329 w345] -> w311
                  tunnel: w308 -> [w321 _]
                  tunnel: w307 -> [w324 _]
                  tunnel: w306 -> [w323 w337]
                  tunnel: [w322 w337] -> w305
                  tunnel: w297 -> [w320 w336]
                  tunnel: w295 -> [_ _]
                  tunnel: w299 -> [w319 w332]
                  tunnel: w296 -> [w317 w331]
                  frame False {
                    n81 = Flatten To JSON(anything=w317, error in (no error)=w319) -> (JSON string=w316:string, 11:w318:errorcluster)  [unwired: 1 in]
                    n82 = call <vilib>:"Unflatten From JSON String.vi"("Type and Defaults"=T15 {"Port"="", "Minor Frame Freq"=0, "Minor Frame Count"=0, "Frame Info"=[], "Sensor Type"=0, "OIM Address"=0} ("Async serial Configuration Cluster"), "error in"=w318, "JSON String"=w316) -> ("error out"=w315:errorcluster, "Variant"=w314:variant)  [unwired: 7 in]
                    n83 = Build Array (concatenate)(w323, w320) -> (w322:string[])
                    n84 = Bundle By Name(cluster=T2 {"State"=enum."Launch Module", "Interface"="AO", "Engine Name"="Slot5_6551_AO", "Varient Data"=variant(string "{"), "SubCmd"="", "Serial Mode"="", "ARINC Board"=0, "Ethernet Mode"=0, "CPU Frequency"=0.0}, "State"=Main_Engine_TCP_Command_Data."Launch Module", "Engine Name"=w320, "Varient Data"=w314, "Interface"=w324, "SubCmd"=w321) -> (w326:T2)
                    n85 = Enqueue Element(queue=w330, element=w326, timeout in ms (-1)=10, error in (no error)=w315) -> (error out=w329:errorcluster)  [unwired: 2 out]
                  }
                  frame True {
                    n86 = Concatenate Strings(w336, "Command Q" ("string")) -> (w344:string)
                    n87 = Obtain Queue(max queue size (-1, unlimited)=10, name (unnamed)=w344, element data type=T18 {"Async serial Configuration Cluster"={"Port"="", "Minor Frame Freq"=0, "Minor Frame Count"=0, "Frame Info"=[], "Sensor Type"=0, "OIM Address"=0}, "Command State"=enum."Configure"}, error in (no error)=w332) -> (queue out=w342:refnum<queue>, error out=w338:errorcluster)  [unwired: 1 in, 1 out]
                    n88 = Bundle By Name(cluster=T18 {"Async serial Configuration Cluster"={"Port"="", "Minor Frame Freq"=0, "Minor Frame Count"=0, "Frame Info"=[], "Sensor Type"=0, "OIM Address"=0}, "Command State"=enum."Configure"}, "Async serial Configuration Cluster"=w331, "Command State"=Main_Engine_JSON_Command_State."Configure") -> (w339:T18)
                    n89 = Enqueue Element(queue=w342, element=w339, timeout in ms (-1)=10, error in (no error)=w338) -> (error out=w345:errorcluster)  [unwired: 2 out]
                  }
                }
              }
              frame "Start" {
                n90 = Concatenate Strings(w346, "Command Q" ("string")) -> (w357:string)
                n91 = Obtain Queue(max queue size (-1, unlimited)=10, name (unnamed)=w357, element data type=T18 {"Async serial Configuration Cluster"={"Port"="", "Minor Frame Freq"=0, "Minor Frame Count"=0, "Frame Info"=[], "Sensor Type"=0, "OIM Address"=0}, "Command State"=enum."Configure"}, error in (no error)=w359) -> (queue out=w355:refnum<queue>, error out=w348:errorcluster)  [unwired: 1 in, 1 out]
                n92 = Bundle By Name(cluster=T18 {"Async serial Configuration Cluster"={"Port"="", "Minor Frame Freq"=0, "Minor Frame Count"=0, "Frame Info"=[], "Sensor Type"=0, "OIM Address"=0}, "Command State"=enum."Configure"}, "Command State"=Main_Engine_JSON_Command_State."Start") -> (w349:T18)
                n93 = Enqueue Element(queue=w355, element=w349, timeout in ms (-1)=10, error in (no error)=w348) -> (error out=w358:errorcluster)  [unwired: 2 out]
              }
              frame "Stop" {
                w367 = T32 {"Stop"=FALSE, "JSON Variant"=variant}
                n94 = Concatenate Strings(w368, "Interupt Q" ("string")) -> (w374:string)
                n95 = Obtain Queue(name (unnamed)=w374, element data type=w367, error in (no error)=w375) -> (queue out=w366:refnum<queue>, error out=w363:errorcluster)  [unwired: 2 in, 1 out]
                n96 = To Variant(anything=T19 {"Port"="", "Message Info"=[]} ("Array")) -> (Variant=w360:variant)
                n97 = Flush Queue(queue=w366, error in (no error)=w363) -> (queue out=w365:refnum<queue>, error out=w364:errorcluster)  [unwired: 1 out]
                n98 = Bundle By Name(cluster=w367, "JSON Variant"=w360, "Stop"=TRUE ("Generation Stop")) -> (w371:T32)
                n99 = Enqueue Element(queue=w365, element=w371, timeout in ms (-1)=10, error in (no error)=w364) -> (error out=w370:errorcluster)  [unwired: 2 out]
              }
              frame "Update" {
                n100 = Number To Decimal String(number=w391) -> (decimal integer string=w389:string)  [unwired: 1 in]
                n101 = Build Array (concatenate)(string[] ["Interface Data", "Data"] ("path"), w389) -> (w377:string[])
                n102 = Unflatten From JSON(path=w377, JSON string=w381, type and defaults=T19 {"Port"="", "Message Info"=[]} ("Array"), error in (no error)=w387) -> (value=w384:T19, error out=w382:errorcluster)  [unwired: 3 in]
                n103 = Concatenate Strings(w386, "Interupt Q" ("string")) -> (w379:string)
                n104 = case shown="No Error" w382 {
                  selector: w382 -> [w403 w410]
                  tunnel: [w408 w416] -> w396
                  tunnel: [w407 w415] -> w395
                  tunnel: [w406 w414] -> w385
                  tunnel: w384 -> [_ w412]
                  tunnel: [w405 w411] -> w383
                  tunnel: w381 -> [w401 _]
                  tunnel: w379 -> [w404 w409]
                  tunnel: T20 {"Port"="", "Pattern"="", "Amplitude"=0.0, "Frequency"=0.0, "Phase"=0, "Sampling info"={"Fs"=1000.0, "#s"=1000.0}} ("Array") -> [w398 _]
                  tunnel: w377 -> [w397 _]
                  frame Error {
                    w406 = T32 {"Stop"=FALSE, "JSON Variant"=variant}
                    n105 = call <vilib>:"Clear Errors.vi"("error in (no error)"=w403) -> ("error out"=w399:errorcluster)  [unwired: 5 in, 1 out]
                    n106 = Unflatten From JSON(path=w397, JSON string=w401, type and defaults=w398, error in (no error)=w399) -> (value=w400:T20, error out=w402:errorcluster)  [unwired: 3 in]
                    n107 = To Variant(anything=w400) -> (Variant=w405:variant)
                    n108 = Obtain Queue(name (unnamed)=w404, element data type=w406, error in (no error)=w402) -> (queue out=w408:refnum<queue>, error out=w407:errorcluster)  [unwired: 2 in, 1 out]
                  }
                  frame No Error {
                    w414 = T32 {"Stop"=FALSE, "JSON Variant"=variant}
                    n109 = To Variant(anything=w412) -> (Variant=w411:variant)
                    n110 = Obtain Queue(max queue size (-1, unlimited)=10, name (unnamed)=w409, element data type=w414, error in (no error)=w410) -> (queue out=w416:refnum<queue>, error out=w415:errorcluster)  [unwired: 1 in, 1 out]
                  }
                }
                n111 = Bundle By Name(cluster=w385, "JSON Variant"=w383) -> (w394:T32)
                n112 = Enqueue Element(queue=w396, element=w394, timeout in ms (-1)=10, error in (no error)=w395) -> (error out=w393:errorcluster)  [unwired: 2 out]
              }
            }
          }
        }
        frame "Ethernet" {
          # "This case handles the functionality of engine launch, configuring the engine & start,stop&update of respective Ethernet communication engines."
          n113 = for {
            tunnel: w424 -> [w435]
            tunnel: w422 -> [w433]
            tunnel: w421 -> [w432]
            tunnel: w417 -> [w431]
            tunnel: w420 -> [w427] mode=indexing
            shift-right: [w437] -> w426
            shift-left: w419 -> [w429]
            tunnel: w418 -> [w430]
            shift-right: [w436] -> w425
            shift-left: w423 -> [w434]
            i -> [w428]
            n114 = case "Command" shown="\"Stop\"" w431 {
              tunnel: w429 -> [w439 w446 w506 w522 w535]
              tunnel: w435 -> [_ w454 _ _ _]
              tunnel: [w439 w453 w505 w517 w540] -> w437
              tunnel: w434 -> [w438 w448 w496 w516 w539]
              tunnel: w433 -> [_ w450 _ _ _]
              tunnel: w432 -> [_ w449 _ _ _]
              tunnel: [w438 w447 w496 w516 w539] -> w436
              tunnel: w430 -> [_ w442 _ _ w530]
              tunnel: w428 -> [_ _ _ _ w538]
              tunnel: w427 -> [_ w444 w495 w515 w534]
              frame Default {
              }
              frame "Configure" {
                n115 = Unflatten From JSON(path=string[] ["Interface Data", "Data"], JSON string=w442, type and defaults=T22 {"Mode"=0, "Local IP"="", "Local Port"=8, "Frame Info"=[], "Minor Frame Freq"=0} ("Ethernet Configuration"), error in (no error)=w446) -> (value=w443:T22, error out=w445:errorcluster)  [unwired: 3 in]
                n116 = Search 1D Array(1D array=w448, element=w444) -> (index of element=w452:i32)  [unwired: 1 in]
                n117 = Greater Or Equal To 0?(x=w452) -> (x >= 0?=w451:bool)
                n118 = case "Engine Active?" shown="False" w451 {
                  tunnel: w454 -> [w477 _]
                  tunnel: [w476 w492] -> w453
                  tunnel: w450 -> [w468 _]
                  tunnel: w449 -> [w471 _]
                  tunnel: w448 -> [w470 w484]
                  tunnel: [w469 w484] -> w447
                  tunnel: w444 -> [w467 w483]
                  tunnel: w442 -> [w458 _]
                  tunnel: w445 -> [w466 w481]
                  tunnel: w443 -> [w465 w478]
                  frame False {
                    n119 = Flatten To JSON(anything=w465, error in (no error)=w466) -> (JSON string=w464:string, 11:w460:errorcluster)  [unwired: 1 in]
                    n120 = Unflatten From JSON(path=string[] ["Interface Data", "Data", "Mode"], JSON string=w458, type and defaults=u8 0 ("Ethernet Mode"), error in (no error)=w460) -> (value=w455:u8, error out=w459:errorcluster)  [unwired: 3 in]
                    n121 = call <vilib>:"Unflatten From JSON String.vi"("Type and Defaults"=T22 {"Mode"=0, "Local IP"="", "Local Port"=8, "Frame Info"=[], "Minor Frame Freq"=0} ("Ethernet Configuration"), "error in"=w459, "JSON String"=w464) -> ("error out"=w463:errorcluster, "Variant"=w462:variant)  [unwired: 7 in]
                    n122 = Build Array (concatenate)(w470, w467) -> (w469:string[])
                    n123 = Bundle By Name(cluster=T2 {"State"=enum."Launch Module", "Interface"="AO", "Engine Name"="Slot5_6551_AO", "Varient Data"=variant(string "{"), "SubCmd"="", "Serial Mode"="", "ARINC Board"=0, "Ethernet Mode"=0, "CPU Frequency"=0.0}, "Ethernet Mode"=w455, "State"=Main_Engine_TCP_Command_Data."Launch Module", "Engine Name"=w467, "Varient Data"=w462, "Interface"=w471, "SubCmd"=w468) -> (w473:T2)
                    n124 = Enqueue Element(queue=w477, element=w473, timeout in ms (-1)=10, error in (no error)=w463) -> (error out=w476:errorcluster)  [unwired: 2 out]
                  }
                  frame True {
                    n125 = Concatenate Strings(w483, "Command Q" ("string")) -> (w491:string)
                    n126 = Obtain Queue(max queue size (-1, unlimited)=10, name (unnamed)=w491, element data type=T26 {"Ethernet Configuration"={"Mode"=0, "Local IP"="", "Local Port"=8, "Frame Info"=[], "Minor Frame Freq"=10}, "Command State"=enum."Configure"} ("Async Serial Command Q Cluster"), error in (no error)=w481) -> (queue out=w489:refnum<queue>, error out=w485:errorcluster)  [unwired: 1 in, 1 out]
                    n127 = Bundle By Name(cluster=T26 {"Ethernet Configuration"={"Mode"=0, "Local IP"="", "Local Port"=8, "Frame Info"=[], "Minor Frame Freq"=10}, "Command State"=enum."Configure"} ("Async Serial Command Q Cluster"), "Ethernet Configuration"=w478, "Command State"=Main_Engine_JSON_Command_State."Configure") -> (w486:T26)
                    n128 = Enqueue Element(queue=w489, element=w486, timeout in ms (-1)=10, error in (no error)=w485) -> (error out=w492:errorcluster)  [unwired: 2 out]
                  }
                }
              }
              frame "Start" {
                n129 = Concatenate Strings(w495, "Command Q" ("string")) -> (w504:string)
                n130 = Obtain Queue(max queue size (-1, unlimited)=10, name (unnamed)=w504, element data type=T26 {"Ethernet Configuration"={"Mode"=0, "Local IP"="", "Local Port"=8, "Frame Info"=[], "Minor Frame Freq"=10}, "Command State"=enum."Configure"} ("Async Serial Command Q Cluster"), error in (no error)=w506) -> (queue out=w502:refnum<queue>, error out=w497:errorcluster)  [unwired: 1 in, 1 out]
                n131 = Bundle By Name(cluster=T26 {"Ethernet Configuration"={"Mode"=0, "Local IP"="", "Local Port"=8, "Frame Info"=[], "Minor Frame Freq"=10}, "Command State"=enum."Configure"} ("Async Serial Command Q Cluster"), "Command State"=Main_Engine_JSON_Command_State."Start") -> (w498:T26)
                n132 = Enqueue Element(queue=w502, element=w498, timeout in ms (-1)=10, error in (no error)=w497) -> (error out=w505:errorcluster)  [unwired: 2 out]
              }
              frame "Stop" {
                w509 = T32 {"Stop"=FALSE, "JSON Variant"=variant} ("Serial Interupt Cluster")
                n133 = Concatenate Strings(w515, "Interupt Q" ("string")) -> (w521:string)
                n134 = To Variant(anything=T27 {"IP"="", "Message Info"=[], "Port"=0} ("Async Update Cluster")) -> (Variant=w507:variant)
                n135 = Obtain Queue(name (unnamed)=w521, element data type=w509, error in (no error)=w522) -> (queue out=w514:refnum<queue>, error out=w511:errorcluster)  [unwired: 2 in, 1 out]
                n136 = Flush Queue(queue=w514, error in (no error)=w511) -> (queue out=w513:refnum<queue>, error out=w512:errorcluster)  [unwired: 1 out]
                n137 = Bundle By Name(cluster=w509, "JSON Variant"=w507, "Stop"=TRUE ("Generation Stop")) -> (w518:T32)
                n138 = Enqueue Element(queue=w513, element=w518, timeout in ms (-1)=10, error in (no error)=w512) -> (error out=w517:errorcluster)  [unwired: 2 out]
              }
              frame "Update" {
                w523 = T32 {"Stop"=FALSE, "JSON Variant"=variant} ("Serial Interupt Cluster")
                n139 = Number To Decimal String(number=w538) -> (decimal integer string=w536:string)  [unwired: 1 in]
                n140 = Build Array (concatenate)(string[] ["Interface Data", "Data"] ("path"), w536) -> (w527:string[])
                n141 = Unflatten From JSON(path=w527, JSON string=w530, type and defaults=T27 {"IP"="", "Message Info"=[], "Port"=0} ("Async Update Cluster"), error in (no error)=w535) -> (value=w533:T27, error out=w531:errorcluster)  [unwired: 3 in]
                n142 = To Variant(anything=w533) -> (Variant=w532:variant)
                n143 = Concatenate Strings(w534, "Interupt Q" ("string")) -> (w528:string)
                n144 = Obtain Queue(max queue size (-1, unlimited)=10, name (unnamed)=w528, element data type=w523, error in (no error)=w531) -> (queue out=w543:refnum<queue>, error out=w542:errorcluster)  [unwired: 1 in, 1 out]
                n145 = Bundle By Name(cluster=w523, "JSON Variant"=w532) -> (w541:T32)
                n146 = Enqueue Element(queue=w543, element=w541, timeout in ms (-1)=10, error in (no error)=w542) -> (error out=w540:errorcluster)  [unwired: 2 out]
              }
            }
          }
        }
        frame "Exit" {
          w550 = T33[] [enum.">Exit"] items=[">Poll", ".........State Machine.........", ">Init", ">Init Configuration", ">Decode Configuration", ">Error", ">Exit", "..........TCP Engine..........", ">Wait for Listener", ">Get Msg from HOST", ">Decode the Command", ">Create Listerner ID"]
          n147 = for {
            tunnel: w545 -> [w565] mode=indexing
            shift-right: [w552] -> _
            shift-left: w544 -> [w555]
            w558 = T8 {"Interface"="AIO", "Interface Data"={"Command"="Configure", "SubCmd"="AO", "Data"=[], "Timing"={"samples per channel"=1000, "sample mode"=10178, "Sampling Rate"=1000.0}}, "Command State"=enum."Configure"} ("AIO Config Cluster")
            w569 = T29 {" Stop"=FALSE, "JSON Variant"=variant(string "")} ("I/O  Interupt Cluster")
            n148 = call <vilib>:"Clear Errors.vi"("error in (no error)"=w555) -> ("error out"=w551:errorcluster)  [unwired: 5 in, 1 out]
            n149 = Concatenate Strings(w565, "Command Q" ("name (unnamed)")) -> (w563:string)
            n150 = Concatenate Strings(w565, "Interupt Q" ("name (unnamed)")) -> (w574:string)
            n151 = Obtain Queue(max queue size (-1, unlimited)=10, name (unnamed)=w563, element data type=w558, error in (no error)=w551) -> (queue out=w561:refnum<queue>, error out=w560:errorcluster)  [unwired: 1 in, 1 out]
            n152 = Obtain Queue(name (unnamed)=w574, element data type=w569, error in (no error)=w551) -> (queue out=w571:refnum<queue>, error out=w570:errorcluster)  [unwired: 2 in, 1 out]
            n153 = Bundle By Name(cluster=w558, "Command State"=Main_Engine_JSON_Command_State."Exit") -> (w557:T8)
            n154 = Flush Queue(queue=w561, error in (no error)=w560) -> (queue out=w562:refnum<queue>, error out=w559:errorcluster)  [unwired: 1 out]
            n155 = Bundle By Name(cluster=w569, "Stop"=TRUE) -> (w568:T29)
            n156 = Flush Queue(queue=w571, error in (no error)=w570) -> (queue out=w573:refnum<queue>, error out=w572:errorcluster)  [unwired: 1 out]
            n157 = Enqueue Element At Opposite End(queue=w573, element=w568, error in (no error)=w572) -> (error out=w553:errorcluster)  [unwired: 1 in, 2 out]
            n158 = Enqueue Element At Opposite End(queue=w562, element=w557, error in (no error)=w559) -> (error out=w554:errorcluster)  [unwired: 1 in, 2 out]
            n159 = Merge Errors(w554, w553) -> (w552:errorcluster)
          }
          n160 = call "TCP Engine SM Q Driver.vi"("Q Driver Options"=TCP_Engine_Q_Driver_Options."Flush Q", "error in"=w544) -> ("error out"=w547:errorcluster)  [unwired: 5 in, 4 out]
          n161 = call "TCP Engine SM Q Driver.vi"("Q Driver Options"=TCP_Engine_Q_Driver_Options."EnQ at Opp", "States"=w550, "error in"=w547) -> ("error out"=w548:errorcluster)  [unwired: 4 in, 4 out]
        }
        frame "General" {
          n162 = case "Command" shown="\"Logging\"" w580 {
            tunnel: [w582 w585 w596] -> w579
            tunnel: w578 -> [w582 w584 w595]
            tunnel: w577 -> [_ w586 w597]
            tunnel: w576 -> [_ w583 w594]
            frame Default {
            }
            frame "AutoSequence" {
              n163 = case "Sub-Command" shown="\"Start\"" w586 {
                tunnel: [w587 w588 w592] -> w585
                tunnel: w584 -> [w587 w589 w593]
                tunnel: w583 -> [_ w590 w591]
                frame Default {
                }
                frame "Configure" {
                  n164 = call "Configuration Data.vi"("error in"=w589, "AS-Configuration Data"=w590) -> ("error out"=w588:errorcluster)  [unwired: 9 in]
                }
                frame "Start" {
                  n165 = call "Start Auto Sequence.vi"("error in"=w593, "Start-AS"=w591) -> ("error out"=w592:errorcluster)  [unwired: 9 in]
                }
              }
            }
            frame "Logging" {
              n166 = case "Sub-Command" shown="\"Configure\"" w597 {
                tunnel: [w598 w604 w605] -> w596
                tunnel: w595 -> [w598 w602 w606]
                tunnel: w594 -> [_ w603 w607]
                frame Default {
                }
                frame "Configure" {
                  n167 = Variant To Data(error in=w602, type=0.0, Variant=w603) -> (data=w599:dbl, error out=w601:errorcluster)
                  n168 = call "Data Logging Duration.vi"("error in"=w601, "Data Logging Duration(Sec)"=w599) -> ("error out"=w604:errorcluster)  [unwired: 9 in]
                }
                frame "Start" {
                  n169 = call "Start Logging.vi"("error in"=w606, "Start Logging"=w607) -> ("error out"=w605:errorcluster)  [unwired: 9 in]
                }
              }
            }
          }
        }
      }
      n170 = Format Into String(format string="Interface %s Command %s SubCmd %s", w18, w17, w16) -> (resulting string=w13:string)  [unwired: 2 in, 1 out]
      n171 = in-place {
        in-place-border: w10 -> [w27]
        n172 = in-place-cluster #1(w12) -> ("source"=w29:string)
        n173 = Concatenate Strings(w27, w29) -> (w28:string)
        n174 = in-place-cluster #1("source"=w28) -> (w11:errorcluster)
      }
      n175 = call "Main Engine Write Data Log File.vi"("error in"=w11, "State"="Send Command to all modules", "Input Data"=w13, "Log file path In"=w14) -> ("error out"=w20:errorcluster)  [unwired: 6 in, 1 out]
    }
    frame Error {
      n176 = in-place {
        in-place-border: w609 -> [w615]
        n177 = in-place-cluster #2(w610) -> ("source"=w616:string)
        n178 = Concatenate Strings(w615, w616) -> (w614:string)
        n179 = in-place-cluster #2("source"=w614) -> (w608:errorcluster)
      }
      n180 = call "Main Engine Write Data Log File.vi"("error in"=w608, "Log file path In"=w611) -> ("error out"=w612:errorcluster)  [unwired: 8 in, 1 out]
    }
  }
  "error out" <- w8
  "Active Engine Names Out" <- w3
